vi "Get Dependent File Property Names.vi"(0 "Device Ref in":T1 format="%.0x", 11 "error in (no error)":errorcluster) -> (4 "Device Ref out":T1 format="%.0x", 6 "driver vi path properties":string[](array[string]), 8 "timing source properties":string[](array[string]), 10 "dependency properties":string[](array[string]), 15 "error out":errorcluster)   [LabVIEW 2026, in "SEECD System Explorer.lvlib"]
uses:
  SEECD System Explorer.lvlib
  <vilib>/NI VeriStand/Custom Device API/Custom Device Item Ref.ctl
  C:/Users/Administrator/Desktop/Jatin/All DNC DLLs/NationalInstruments.VeriStand.SystemDefinitionAPI.dll
  Jatin/All DNC DLLs/NationalInstruments.VeriStand.SystemDefinitionAPI.dll
  C:/Users/Administrator/Desktop/Jatin/All DNC DLLs/NationalInstruments.VeriStand.SystemStorage.dll
  Jatin/All DNC DLLs/NationalInstruments.VeriStand.SystemStorage.dll
  <vilib>/NI VeriStand/Custom Device API/Custom Device API.lvlib
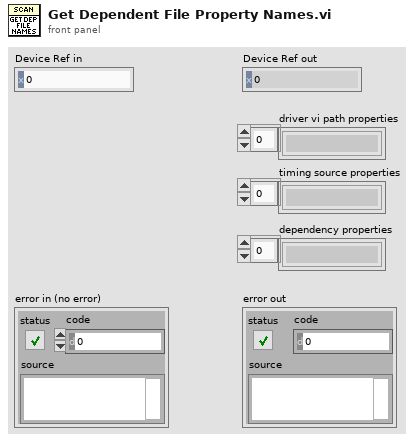
[diagram p1: front panel]
types:
  T1 = typedef "Custom Device API.lvlib/Custom Device Item Ref.ctl" = u64
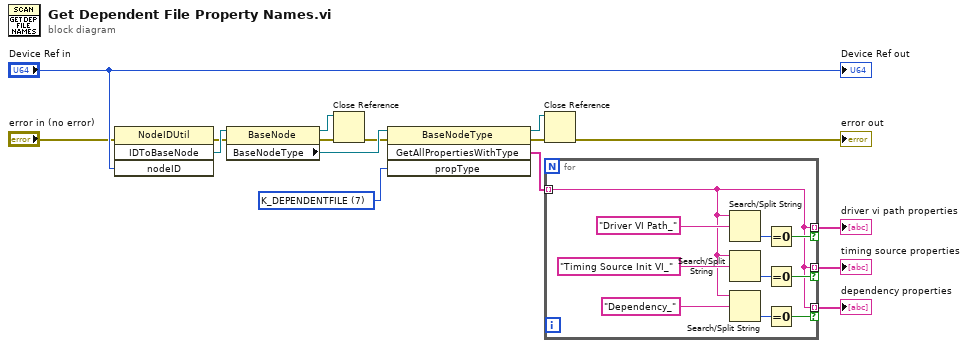
[diagram p0: block diagram]
diagram:
  w16 = 7 items=["K_STRING", "K_BOOL", "K_I32", "K_U32", "K_DOUBLE", "K_U64", "K_VARIANT", "K_DEPENDENTFILE", "K_DEPENDENTNODE", "K_DATASOURCENODE", "K_U16", "K_DBLARR", "K_U32ARR", "K_I32ARR", "K_STRINGARR", "K_DICTIONARY", "K_DICTIONARYARR", "K_BINARYSTRING", "K_I16", "K_I64", "K_BOOLARR", "K_U64ARR", "K_U16ARR", "K_I64ARR", "K_I16ARR"] ("propType")
  n1 = invoke class="NodeIDUtil" method="IDToBaseNode"(error in="error in (no error)", "nodeID"="Device Ref in") -> (error out=w9:errorcluster, "IDToBaseNode"=w14:refnum<k39>)  [unwired: 2 in, 2 out]
  n2 = property class="BaseNode"(reference=w14, error in=w9) -> (reference out=w11:refnum<k39>, error out=w10:errorcluster, "BaseNodeType"=w15:refnum<k39>)
  n3 = Close Reference(reference=w11, error in (no error)=w10) -> (error out=w8:errorcluster)
  n4 = invoke class="BaseNodeType" method="GetAllPropertiesWithType"(reference=w15, error in=w8, "propType"=w16) -> (reference out=w6:refnum<k39>, error out=w7:errorcluster, "GetAllPropertiesWithType"=w12:string[])  [unwired: 1 in, 1 out]
  n5 = Close Reference(reference=w6, error in (no error)=w7) -> (error out=→"error out":errorcluster)
  n6 = for {
    tunnel: w12 -> [w17] mode=indexing
    tunnel: [w17] -> w3 mode=indexing if=w25
    tunnel: [w17] -> w2 mode=indexing if=w24
    tunnel: [w17] -> w1 mode=indexing if=w21
    n7 = Search/Split String(string=w17, search string/char (-)="Driver VI Path_") -> (offset of match=w23:i32)  [unwired: 1 in, 2 out]
    n8 = Search/Split String(string=w17, search string/char (-)="Timing Source Init VI_") -> (offset of match=w26:i32)  [unwired: 1 in, 2 out]
    n9 = Search/Split String(string=w17, search string/char (-)="Dependency_") -> (offset of match=w22:i32)  [unwired: 1 in, 2 out]
    n10 = Equal To 0?(x=w23) -> (x = 0?=w24:bool)
    n11 = Equal To 0?(x=w26) -> (x = 0?=w25:bool)
    n12 = Equal To 0?(x=w22) -> (x = 0?=w21:bool)
  }
  "dependency properties" <- w1
  "timing source properties" <- w3
  "driver vi path properties" <- w2
  "Device Ref out" <- "Device Ref in"
